vi "OverlayFreezeRange.vi"(1 "FreezeIdx":i32[](array[numeric]), 2 "FreezeArray":bool[](array[boolean])) -> (0 "Range":i32)   [LabVIEW 2022 SP3]
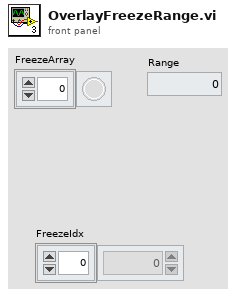
[diagram p1: front panel]
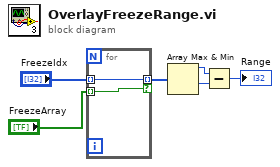
[diagram p0: block diagram]
diagram:
  n1 = for {
    tunnel: "FreezeIdx" -> [w8] mode=indexing
    tunnel: [w8] -> w4 mode=indexing if=w7
    tunnel: "FreezeArray" -> [w7] mode=indexing
  }
  n2 = Array Max & Min(array=w4) -> (max value=w3:i32, min value=w2:i32)  [unwired: 2 out]
  n3 = Subtract(x=w3, y=w2) -> (x-y=→"Range":i32)
